vi "ConvertPotentiometerToDegrees.vi"(2 "Calibration Angle (deg)":dbl, 4 "Potentiometer Calibration Value [0-1]":dbl, 6 "Raw Potentiometer Value [0,1]":dbl) -> (0 "Orientation (deg) [-180,+180]":dbl)   [LabVIEW 2020]
doc: "Converts a potentiometer (or similar analog sensor) from a range of 0 to 1, to -180 degrees to +180 degrees. Supports a calibration value at an arbitrary angle."
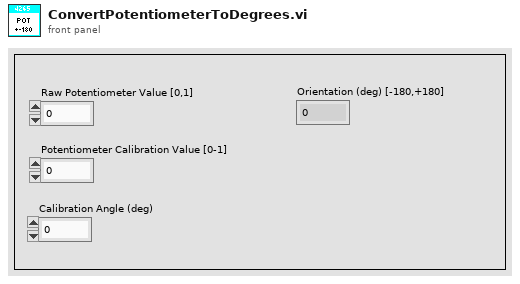
[diagram p1: front panel]
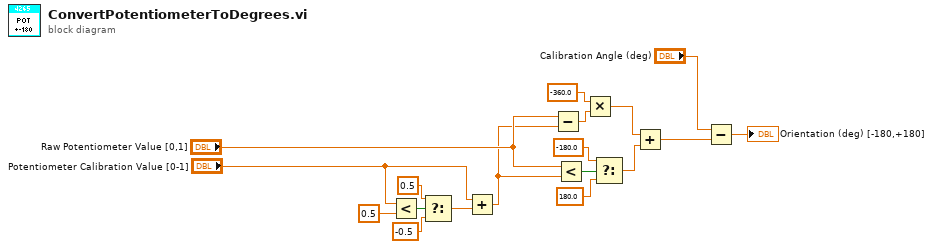
[diagram p0: block diagram]
diagram:
  n1 = Less?(x="Potentiometer Calibration Value [0-1]", y=0.5) -> (x < y?=w13:bool)
  n2 = Select(t=0.5 ("x"), s=w13, f=-0.5 ("x")) -> (s? t:f=w16:dbl)
  n3 = Add(x="Potentiometer Calibration Value [0-1]", y=w16) -> (x+y=w11:dbl)
  n4 = Subtract(x="Raw Potentiometer Value [0,1]", y=w11) -> (x-y=w5:dbl)
  n5 = Less?(x="Raw Potentiometer Value [0,1]", y=w11) -> (x < y?=w10:bool)
  n6 = Multiply(x=-360.0, y=w5) -> (x*y=w6:dbl)
  n7 = Select(t=-180.0, s=w10, f=180.0) -> (s? t:f=w7:dbl)
  n8 = Add(x=w6, y=w7) -> (x+y=w1:dbl)
  n9 = Subtract(x="Calibration Angle (deg)", y=w1) -> (x-y=→"Orientation (deg) [-180,+180]":dbl)
